vi "StealCan.vi"(10 "HMI to Control":T1, 11 "SensorInputData":T2) -> (2 "HMI to ControlOut":T1, 3 "SensorInputDataOut":T2, 4 "Done":bool=TRUE)   [LabVIEW 2015]
uses:
  Typedefs/SensorInputData.ctl
  Typedefs/HMI_to_Control.ctl
panel:
  in  "arguments":string[](array[string])
  in  "dt":i32
  in  "Reinit":bool
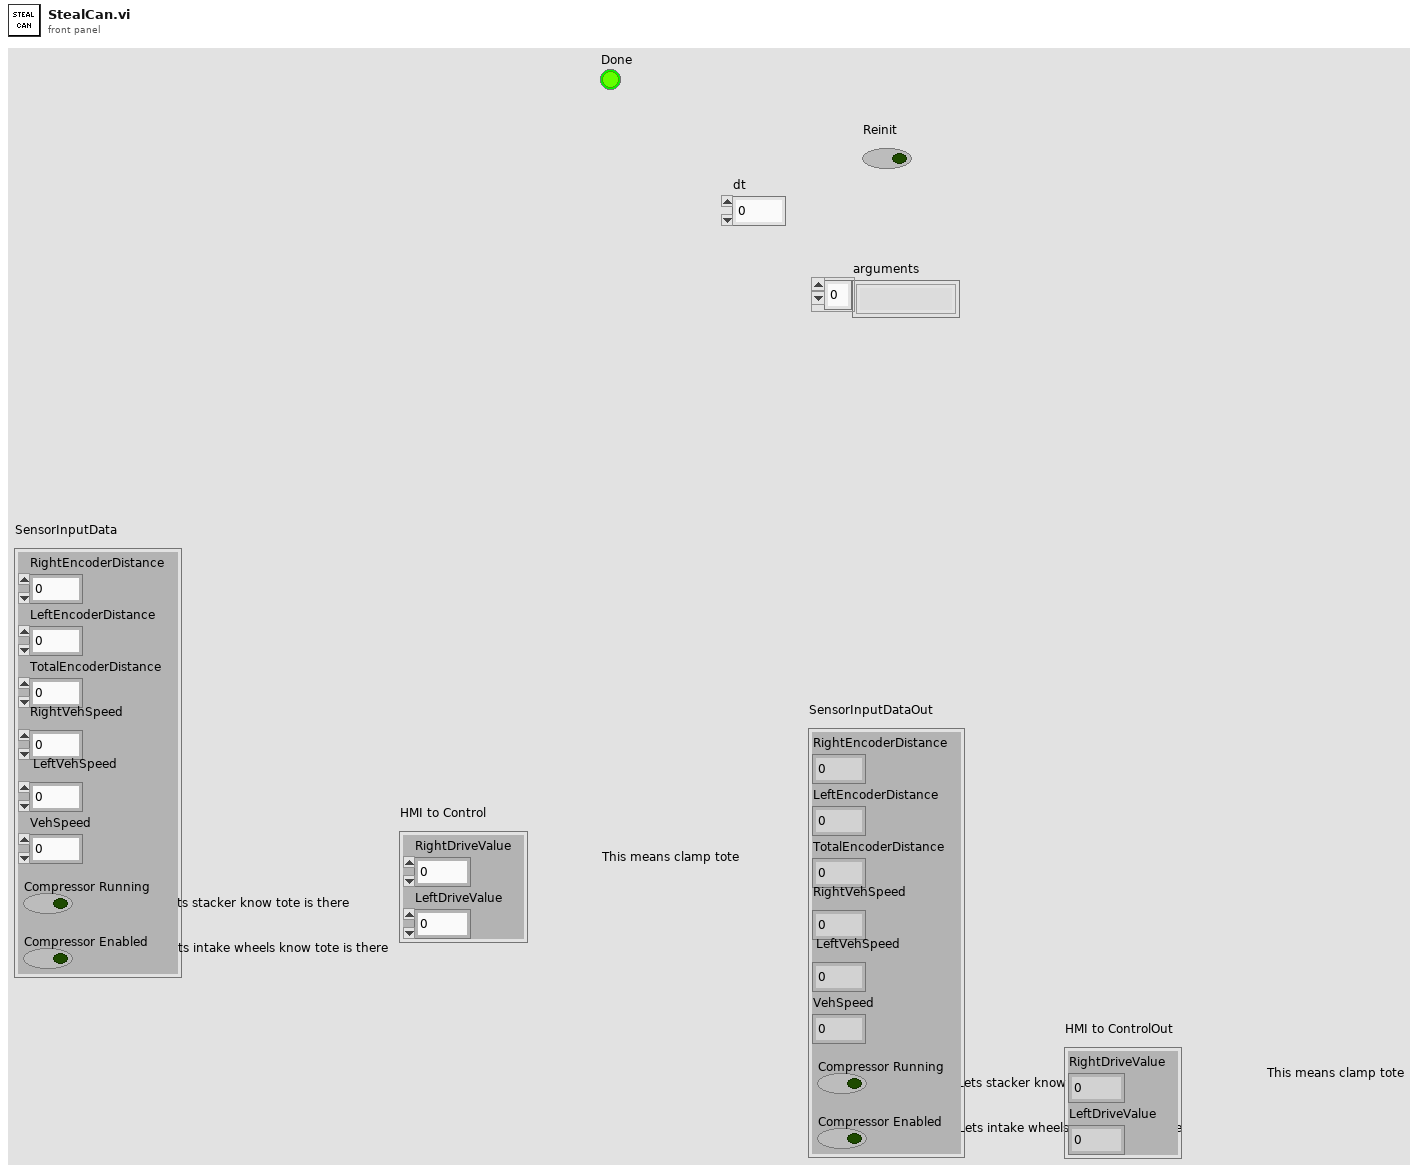
[diagram p1: front panel]
types:
  T1 = typedef "HMI_to_Control.ctl" = cluster{"RightDriveValue":dbl, "LeftDriveValue":dbl}
  T2 = typedef "SensorInputData.ctl" = cluster{"RightEncoderDistance":dbl, "LeftEncoderDistance":dbl, "TotalEncoderDistance":dbl, "RightVehSpeed":dbl, "LeftVehSpeed":dbl, "VehSpeed":dbl, "Compressor Running":bool, "Compressor Enabled":bool}
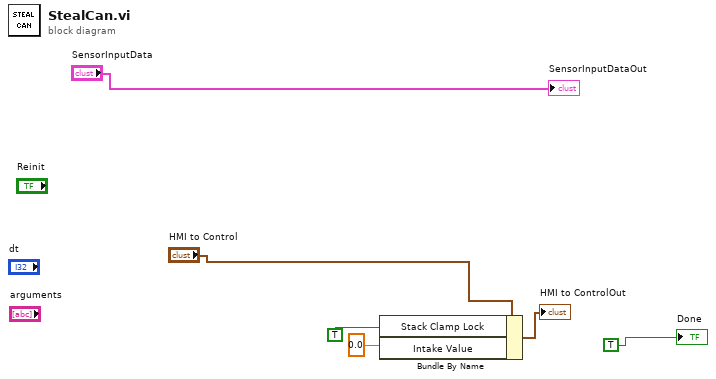
[diagram p0: block diagram]
diagram:
  n1 = Bundle By Name(cluster="HMI to Control", "Stack Clamp Lock"=TRUE ("Inver. Wheels  In Request"), "Intake Value"=sgl 0.0) -> (→"HMI to ControlOut":T1)
  "SensorInputDataOut" <- "SensorInputData"
  "Done" <- TRUE
